vi "trio_stepper_axis.vi"(11 "Encoder axis":i32) -> (3 "Stepper axis":i32)   [LabVIEW 2017]
panel:
  # "With the Trio controller we have encoder input on axes 0-3 and outputs on 4-7"
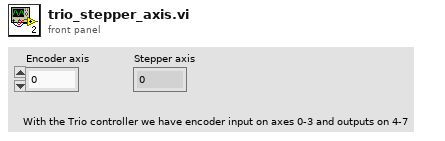
[diagram p1: front panel]
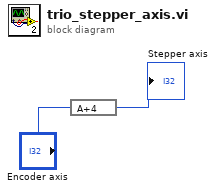
[diagram p0: block diagram]
diagram:
  n1 = expression code="A+4"("Encoder axis") -> (→"Stepper axis":i32)
